vi "Get Thermometer Calibration.vi"() -> (0 "Cancelled":bool, 1 "Thermometer Calibration Data":dbl[][](array[numeric]) format="%.2f", 2 "ID String":string)   [LabVIEW 2021]
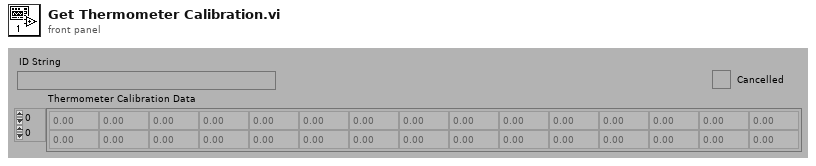
[diagram p1: front panel]
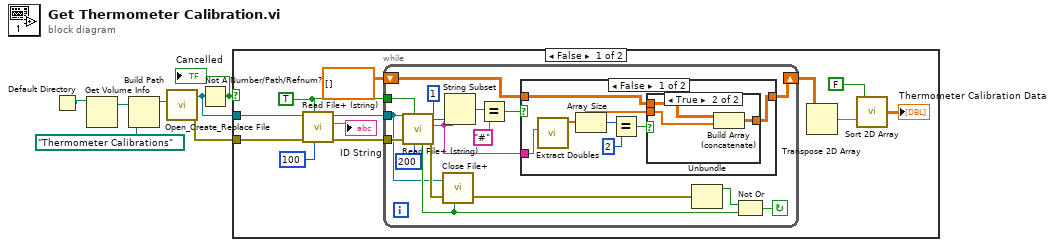
[diagram p0: block diagram]
diagram:
  n1 = Default Directory() -> (w6:path)
  n2 = Get Volume Info(11:w6) -> (5:w5:path)  [unwired: 1 in, 5 out]
  n3 = Build Path(base path=w5, name or relative path=path "Thermometer Calibrations") -> (appended path=w4:path)
  n4 = call <vilib>:"Open_Create_Replace File.vi"("start path  (Not A Path)"=w4) -> ("error out"=w1:errorcluster, "refnum"=w2:refnum<file>)  [unwired: 7 in, 2 out]
  n5 = Not A Number/Path/Refnum?(number/path/refnum=w2) -> (NaN/Path/Refnum?=w3:bool)
  "Cancelled" <- w3
  n6 = case shown="False" w3 {
    tunnel: w2 -> [w10 _]
    tunnel: w1 -> [w19 _]
    frame False {
      w15 = TRUE
      n7 = call <vilib>:"Read File+ (string).vi"("count"=100, "line mode (characters:F)"=w15, "error in (no error)"=w19, "refnum"=w10) -> ("error out"=w18:errorcluster, "string"=→"ID String":string, "dup refnum"=w17:refnum<file>)  [unwired: 3 in, 2 out]
      n8 = while {
        shift-left: dbl[][] [] -> [w22]
        shift-right: [w21] -> w11
        tunnel: w15 -> [w27]
        tunnel: w18 -> [w28]
        tunnel: w17 -> [w23]
        stop <- w29 continue-if-true
        n9 = call <vilib>:"Read File+ (string).vi"("count"=200, "line mode (characters:F)"=w27, "error in (no error)"=w28, "refnum"=w23) -> ("error out"=w25:errorcluster, "string"=w31:string, "EOF?"=w24:bool)  [unwired: 3 in, 2 out]
        n10 = call <vilib>:"Close File+.vi"("error in (no error)"=w25, "close when? (now:T)"=w24, "refnum"=w23) -> ("error out"=w26:errorcluster)  [unwired: 2 in, 2 out]
        n11 = String Subset(string=w31, length (rest)=1) -> (substring=w35:string)  [unwired: 1 in]
        n12 = Equal?(x=w35, y="#") -> (x = y?=w32:bool)
        n13 = case shown="False" w32 {
          tunnel: w31 -> [w36 _]
          tunnel: w22 -> [w38 w47]
          tunnel: [w37 w47] -> w21
          frame False {
            n14 = call "Extract Doubles.vi"("String"=w36) -> ("Data"=w42:dbl[])  [unwired: 5 in, 1 out]
            n15 = Array Size(array=w42) -> (size(s)=w41:i32)
            n16 = Equal?(x=w41, y=2) -> (x = y?=w39:bool)
            n17 = case shown="True" w39 {
              tunnel: w42 -> [_ w44]
              tunnel: [w43 w46] -> w37
              tunnel: w38 -> [w43 w45]
              frame False {
              }
              frame True {
                n18 = Build Array (concatenate)(w45, w44) -> (w46:dbl[][])
              }
            }
          }
          frame True {
          }
        }
        n19 = Unbundle(w26) -> ("status"=w30:bool)  [unwired: 2 out]
        n20 = Not Or(1:w24, 2:w30) -> (0:w29:bool)
      }
      n21 = Transpose 2D Array(2D array=w11) -> (transposed array=w13:dbl[][])
      n22 = call "Sort 2D Array.vi"(1:w13, "First Column"=FALSE) -> (0:→"Thermometer Calibration Data":dbl[][])
    }
    frame True {
    }
  }
